vi "4bar Contol Loop.vi"() -> ()   [LabVIEW 2018]
uses:
  <vilib>/Rock Robotics/WPI/ThirdParty/Phoenix-LabVIEW/Motor Controller/Controls/CTRE_Phoenix_MotorControl_NeutralMode.ctl
  Infrastructure/RobotMap.vi
  Infrastructure/Constants.vi
  <vilib>/Rock Robotics/WPI/Switch/WPI_SwitchOpenLimit.vi
  Robot Global Data.vi
  <vilib>/Rock Robotics/WPI/ThirdParty/Phoenix-LabVIEW/Motor Controller/Get/CTRE_Phoenix_MotorController_GetSelectedSensorData.vi
panel:
  out "4bar Velocity":i32(graph)
  out "4bar Position":i32(graph)
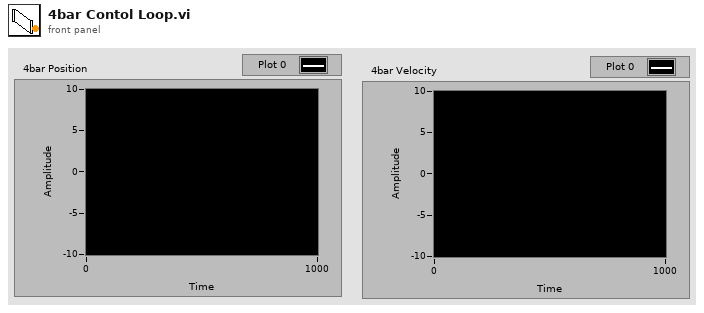
[diagram p1: front panel]
types:
  T1 = typedef "CTRE_Phoenix_MotorControl_NeutralMode.ctl" = enum8{"EEPROMSetting", "Override to Coast", "Override to Brake"}
  T2 = typedef "WPI_MotorControlDeviceRef.ctl" = cluster{"DeviceStatus":errorcluster, "Type":T3, "PWM":cluster{"PWM Channel":T4, "DeadBand":T5}, "CAN":cluster{"Device Number":u8, "SetOutput VI Ref":variant, "GetOutput VI Ref":variant, "Enable VI Ref":variant, "Disable VI Ref":variant, "Data":variant}, "Invert":bool, "DIO PWM":cluster{"PWM \"Enable\" Channel":T4, "DIOChannel":T6, "PWM Rate":dbl}}
  T3 = typedef "WPI_MotorControlType.ctl" = enum16{"PWM", "CAN", "DIO PWM"}
  T4 = typedef "FPGA_DIOPWMChannel.ctl" = enum8{"PWM 0", "PWM 1", "PWM 2", "PWM 3", "PWM 4", "PWM 5", "PWM 6", "PWM 7", "PWM 8", "PWM 9", "PWM MXP 0", "PWM MXP 1", "PWM MXP 2", "PWM MXP 3", "PWM MXP 4", "PWM MXP 5", "PWM MXP 6", "PWM MXP 7", "PWM MXP 8", "PWM MXP 9", "Invalid"}
  T5 = typedef "WPI_PWMDeadband.ctl" = cluster{"Name":string, "maxPositivePwm":i32, "minPositivePwm":i32, "centerPwm":i32, "maxNegativePwm":i32, "minNegativePwm":i32, "angularRange":u16}
  T6 = typedef "FPGA_DIOChannel.ctl" = enum8{"DIO 0", "DIO 1", "DIO 2", "DIO 3", "DIO 4", "DIO 5", "DIO 6", "DIO 7", "DIO 8", "DIO 9", "DIO MXP 0", "DIO MXP 1", "DIO MXP 2", "DIO MXP 3", "DIO MXP 4", "DIO MXP 5", "DIO MXP 6", "DIO MXP 7", "DIO MXP 8", "DIO MXP 9", "DIO MXP 10", "DIO MXP 11", "DIO MXP 12", "DIO MXP 13", "DIO MXP 14", "DIO MXP 15", "SPI Port CS1", "SPI Port CS2", "SPI Port CS3", "SPI Port MISO", "SPI Port MOSI", "Invalid"}
  T7 = typedef "WPI_SwitchDevRef.ctl" = cluster{"DevStatus":errorcluster, "DIO Channel":T6, "CntIndex":T8, "Normally Closed":bool}
  T8 = typedef "FPGA_CounterCtrSystemIndex.ctl" = enum8{"Ctr 0", "Ctr 1", "Ctr 2", "Ctr 3", "Ctr 4", "Ctr 5", "Ctr 6", "Ctr 7", "Invalid"}
  T9 = cluster{"P":dbl, "I":dbl, "D":dbl, "F":dbl, "I Zone":dbl}
  T10 = cluster{"Cruise Velocity":i32, "Acceleration":i32}
  T11 = typedef "CTRE_Phoenix_MotorControl_ControlMode.ctl" = u16
  T12 = cluster{"Control Mode":T11, "Operator Right Joystick Y out":dbl}
  T13 = cluster{"Position (Raw Sensor Units)":i32, "Velocity (Raw Sensor Units per 100 ms)":i32}
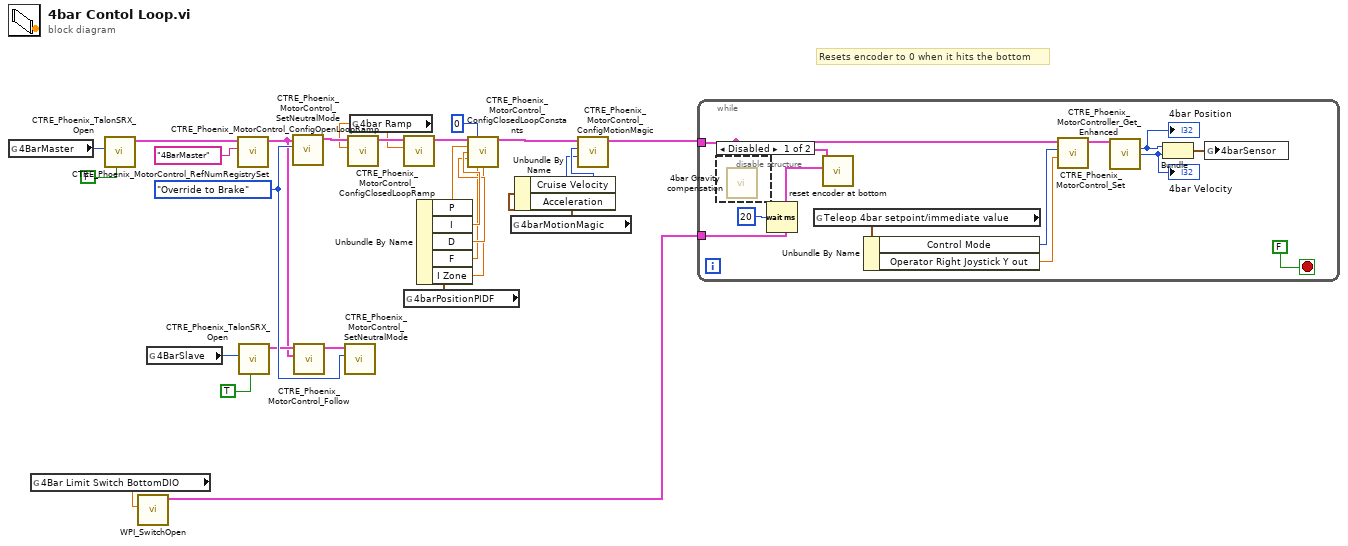
[diagram p0: block diagram]
diagram:
  w28 = CTRE_Phoenix_MotorControl_NeutralMode."Override to Brake" ("Motor Control Neutral Mode")
  # "Resets encoder to 0 when it hits the bottom"
  n1 = global read "RobotMap.vi" "4BarMaster"() -> (w20:u8)
  n2 = global read "RobotMap.vi" "4Bar Limit Switch BottomDIO"() -> (w21:dbl)
  n3 = call <vilib>:"CTRE_Phoenix_TalonSRX_Open.vi"("Invert"=FALSE, "Device Number"=w20) -> ("CAN Talon SRX Ref"=w25:T2)  [unwired: 8 in, 1 out]
  n4 = call-poly <vilib>:"WPI_SwitchOpen.vi"("DIO Channel"=w21) -> ("SwitchDevRef"=w22:T7)  [unwired: 9 in, 1 out]
  n5 = global read "RobotMap.vi" "4BarSlave"() -> (w19:u8)
  n6 = call <vilib>:"CTRE_Phoenix_MotorControl_RefNumRegistrySet.vi"("refnum name"="4BarMaster", "PhoenixMotorControlDevRef"=w25) -> ("PhoenixMotorControlDevRef"=w8:T2)  [unwired: 8 in, 1 out]
  n7 = call <vilib>:"CTRE_Phoenix_TalonSRX_Open.vi"("Invert"=TRUE, "Device Number"=w19) -> ("CAN Talon SRX Ref"=w23:T2)  [unwired: 8 in, 1 out]
  n8 = call <vilib>:"CTRE_Phoenix_MotorControl_SetNeutralMode.vi"("Motor Control Neutral Mode"=w28, "PhoenixMotorControlDevRef"=w8) -> ("PhoenixMotorControlDevRef"=w24:T2)  [unwired: 8 in, 1 out]
  n9 = call <vilib>:"CTRE_Phoenix_MotorControl_Follow.vi"("Master Controller to Follow"=w8, "PhoenixMotorControlDevRef"=w23) -> ("PhoenixMotorControlDevRef"=w27:T2)  [unwired: 8 in, 1 out]
  n10 = call <vilib>:"CTRE_Phoenix_MotorControl_SetNeutralMode.vi"("Motor Control Neutral Mode"=w28, "PhoenixMotorControlDevRef"=w27) -> ()  [unwired: 8 in, 2 out]
  n11 = global read "Constants.vi" "4bar Ramp"() -> (w17:dbl)
  n12 = call <vilib>:"CTRE_Phoenix_MotorControl_ConfigOpenLoopRamp.vi"("secondsFromNeutralToFull"=w17, "PhoenixMotorControlDevRef"=w24) -> ("PhoenixMotorControlDevRef"=w18:T2)  [unwired: 8 in, 1 out]
  n13 = call <vilib>:"CTRE_Phoenix_MotorControl_ConfigClosedLoopRamp.vi"("secondsFromNeutralToFull"=w17, "PhoenixMotorControlDevRef"=w18) -> ("PhoenixMotorControlDevRef"=w10:T2)  [unwired: 8 in, 1 out]
  n14 = global read "Constants.vi" "4barPositionPIDF"() -> (w16:T9)
  n15 = Unbundle By Name(w16) -> ("P"=w15:dbl, "I"=w14:dbl, "D"=w13:dbl, "F"=w12:dbl, "I Zone"=w11:dbl)
  n16 = call <vilib>:"CTRE_Phoenix_MotorControl_ConfigClosedLoopConstants.vi"("PhoenixMotorControlDevRef"=w10, "slotIdx"=0, "P"=w15, "I"=w14, "D"=w13, "F"=w12, "I Zone"=w11) -> ("PhoenixMotorControlDevRef"=w5:T2)  [unwired: 7 in, 1 out]
  n17 = global read "Constants.vi" "4barMotionMagic"() -> (w3:T10)
  n18 = Unbundle By Name(w3) -> ("Cruise Velocity"=w2:i32, "Acceleration"=w1:i32)
  n19 = call <vilib>:"CTRE_Phoenix_MotorControl_ConfigMotionMagic.vi"("Acceleration"=w1, "Cruise Velocity"=w2, "PhoenixMotorControlDevRef"=w5) -> ("PhoenixMotorControlDevRef"=w4:T2)  [unwired: 7 in, 1 out]
  n20 = while {
    tunnel: w4 -> [w29]
    tunnel: w22 -> [w36]
    stop <- FALSE stop-if-true
    n21 = disable-structure shown="Disabled" {
      frame Disabled {
        n22 = call "4bar Gravity compensation.vi"() -> ()  [unwired: 11 in, 1 out]
      }
      frame Enabled {
      }
    }
    n23 = Wait (ms)(milliseconds to wait=u32 20) -> ()  [unwired: 1 out]
    n24 = global read "Robot Global Data.vi" "Teleop 4bar setpoint/immediate value"() -> (w32:T12)
    n25 = call "reset encoder at bottom.vi"("Limit Switch"=w36, "PhoenixMotorControlDevRef"=w29) -> ()  [unwired: 9 in, 1 out]
    n26 = Unbundle By Name(w32) -> ("Control Mode"=w37:T11, "Operator Right Joystick Y out"=w33:dbl)
    n27 = call <vilib>:"CTRE_Phoenix_MotorControl_Set.vi"("Output"=w33, "Control Mode"=w37, "PhoenixMotorControlDevRef"=w29) -> ("PhoenixMotorControlDevRef"=w35:T2)  [unwired: 7 in, 1 out]
    n28 = call-poly <vilib>:"CTRE_Phoenix_MotorController_Get_Enhanced.vi"("PhoenixMotorControlDevRef"=w35) -> ("Position (Raw Sensor Units)"=w31:i32, "Velocity (Raw Sensor Units per 100 ms)"=w30:i32)  [unwired: 11 in, 2 out]
    "4bar Position" <- w31
    "4bar Velocity" <- w30
    n29 = Bundle("Position (Raw Sensor Units)"=w31, "Velocity (Raw Sensor Units per 100 ms)"=w30) -> (w34:T13)  [unwired: 1 in]
    n30 = global write "Robot Global Data.vi" "4barSensor"(w34) -> ()
  }
